vi "Get VF Setpoints.vi"(10 "Per-Unitized VF Voltage Setpoint":dbl, 11 "Generic Optimization in":refnum<class "Generic Optimization.lvclass">) -> (1 "VF Frequency Setpoint":dbl, 2 "VF Voltage Setpoint":dbl, 3 "Generic Optimization out":refnum<class "Generic Optimization.lvclass">)   [LabVIEW 2018, in "Generic Optimization Actor.lvlib" / "Generic Optimization.lvclass"]
uses:
  Generic Optimization.lvclass
  C:/Users/Administrator/Desktop/2018LabVIEW EMS/EMS Generic Actor/EMS Generic/EMS Generic.lvclass
  EMS Generic Actor/EMS Generic/EMS Generic.lvclass
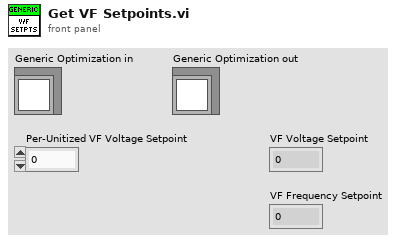
[diagram p1: front panel]
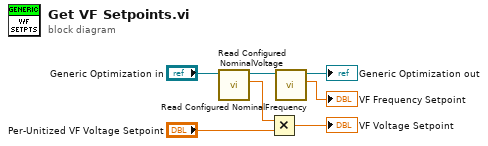
[diagram p0: block diagram]
diagram:
  n1 = call "Read Configured NominalVoltage.vi"("EMS Generic in"="Generic Optimization in") -> ("NominalVoltage"=w1:dbl, "EMS Generic out"=w6:refnum<class "Generic Optimization.lvclass">)  [unwired: 8 in, 1 out]
  n2 = Multiply(x=w1, y="Per-Unitized VF Voltage Setpoint") -> (x*y=→"VF Voltage Setpoint":dbl)
  n3 = call "Read Configured NominalFrequency.vi"("EMS Generic in"=w6) -> ("NominalFrequency"=→"VF Frequency Setpoint":dbl, "EMS Generic out"=→"Generic Optimization out":refnum<class "Generic Optimization.lvclass">)  [unwired: 8 in, 1 out]
